vi "Set Log File Type.vi"(8 "error in (no error)":errorcluster, 10 "Log File Type":T1, 11 "Log File in":refnum<class "Log File.lvclass">) -> (0 "error out":errorcluster, 3 "Log File out":refnum<class "Log File.lvclass">)   [LabVIEW 2015, in "Log File.lvclass"]
uses:
  Log File.lvclass
  Log File Type.ctl
  Log File.lvclass/Log File.ctl
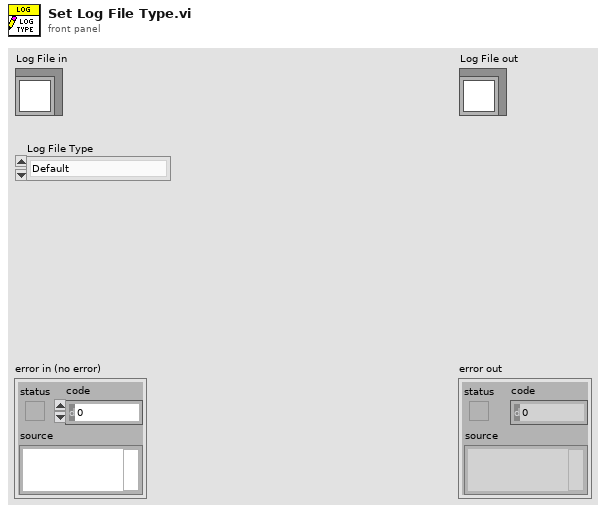
[diagram p1: front panel]
types:
  T1 = typedef "Log File.lvclass/Log File Type.ctl" = enum16{"Default", "TDMS", "Text"}
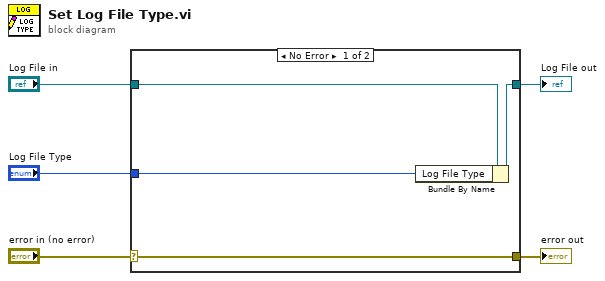
[diagram p0: block diagram]
diagram:
  n1 = case shown="No Error" "error in (no error)" {
    selector: "error in (no error)" -> [w9 w10]
    tunnel: [w9 w10] -> w4
    tunnel: [w7 w11] -> w2
    tunnel: "Log File in" -> [w8 w11]
    tunnel: "Log File Type" -> [w6 _]
    frame No Error {
      n2 = Bundle By Name(cluster=w8, "Log File Type"=w6) -> (w7:refnum<class "Log File.lvclass">)
    }
    frame Error {
    }
  }
  "error out" <- w4
  "Log File out" <- w2
